vi "HW DIY.vi"() -> ()   [LabVIEW 2015]
panel:
  in  "stop":bool
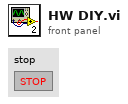
[diagram p1: front panel]
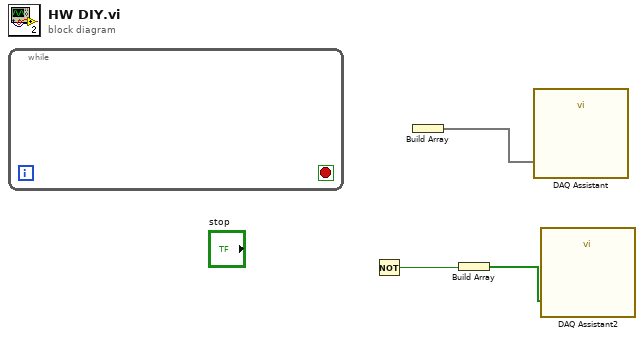
[diagram p0: block diagram]
diagram:
  n1 = while {
    stop <- _ stop-if-true
  }
  n2 = Not() -> (.not. x?=w1:bool)  [unwired: 1 in]
  n3 = Build Array() -> (w3:void[])  [unwired: 1 in]
  n4 = Build Array(w1) -> (w2:bool[])
  n5 = call "DAQ Assistant"("data"=w3) -> ()  [unwired: 17 in, 2 out]
  n6 = call "DAQ Assistant2"("data"=w2) -> ()  [unwired: 17 in, 2 out]
